vi "Reports.vi"() -> ()   [LabVIEW 2017]
uses:
  Globle/Breakdown Rep.vi
  Globle/Trigger Home Screen.vi
panel:
  out "appended array":refnum<vi>[](array[refnum])
  in  "Cancel Button\n- Archive":bool
  in  "Rej Cnt":bool
  in  "OEE":bool
  in  "PC Hr":bool
  in  "PC Day":bool
  in  "Para Report":bool
  in  "PC Month":bool
  in  "BD Day":bool
  in  "BD Yr":bool
  in  "BD Month":bool
  in  "BD MAnage":bool
  in  "BD Action Taken":bool
  in  "BD Analysis":bool
  # "Reports"
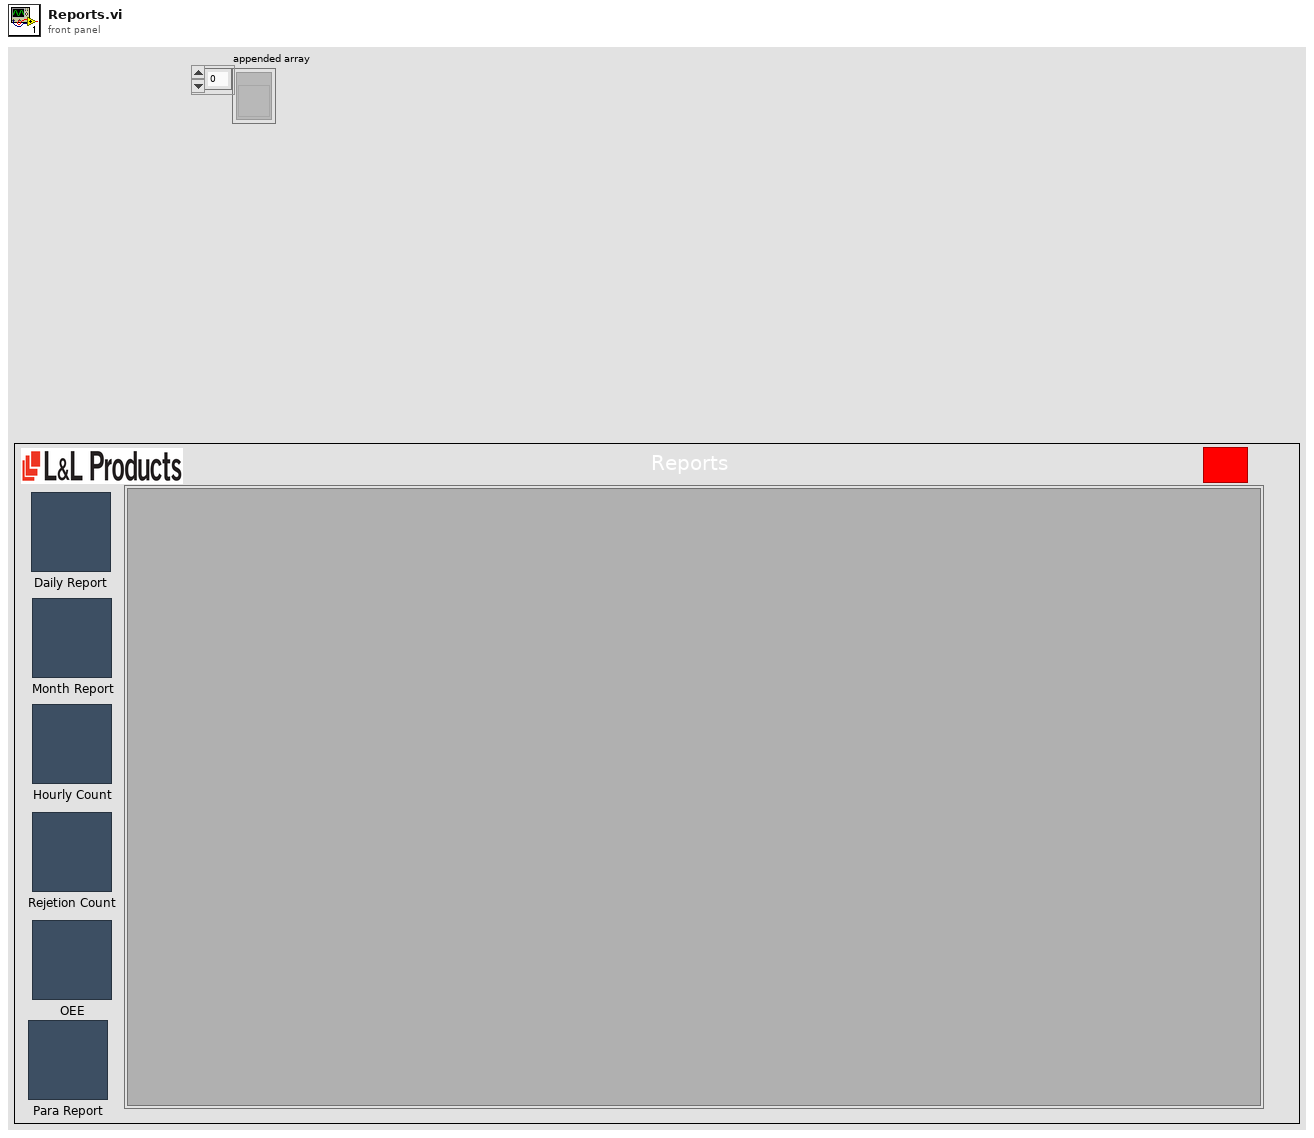
[diagram p1: front panel]
types:
  T1 = enum32{"invalid app kind", "Development System", "Run Time System", "Student Edition", "Embedded LabVIEW", "Evaluation", "Custom"}
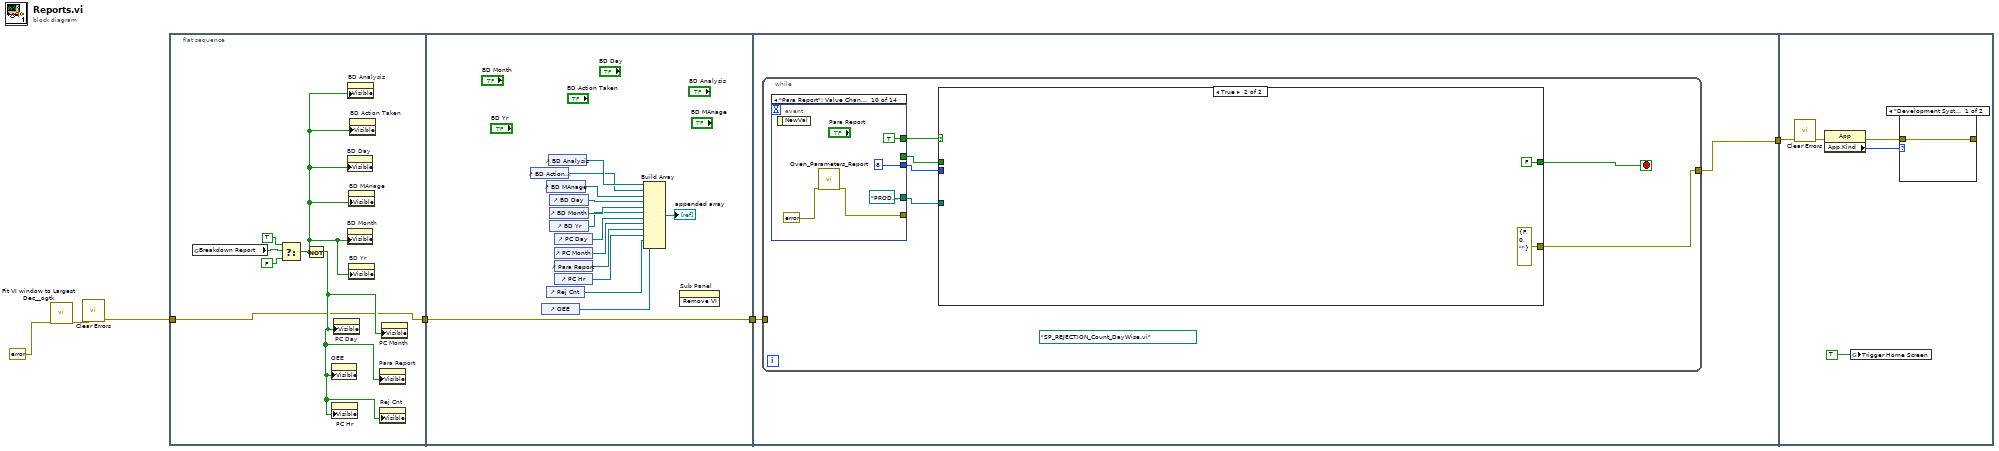
[diagram p0: block diagram]
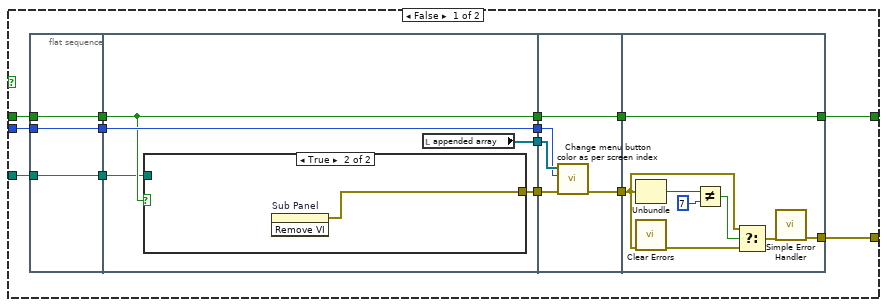
[diagram p2: hidden frame]
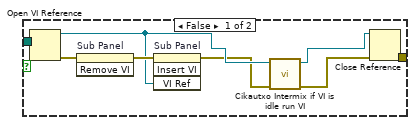
[diagram p3: hidden frame]
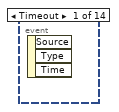
[diagram p4: hidden frame]
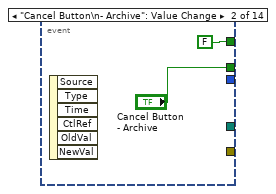
[diagram p5: hidden frame]
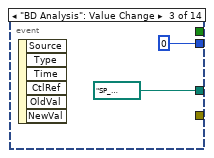
[diagram p6: hidden frame]
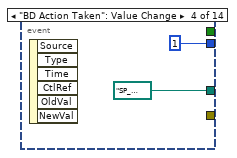
[diagram p7: hidden frame]
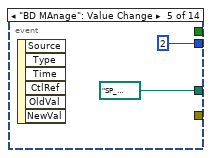
[diagram p8: hidden frame]
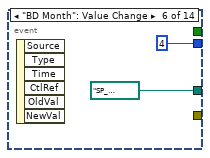
[diagram p9: hidden frame]
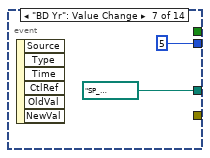
[diagram p10: hidden frame]
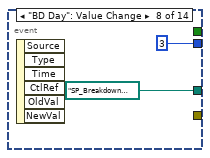
[diagram p11: hidden frame]
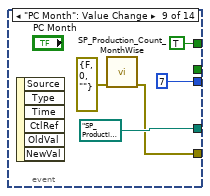
[diagram p12: hidden frame]
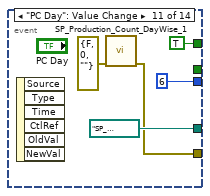
[diagram p13: hidden frame]
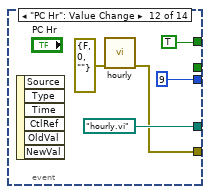
[diagram p14: hidden frame]
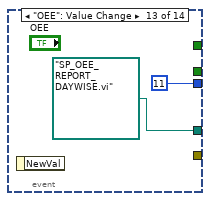
[diagram p15: hidden frame]
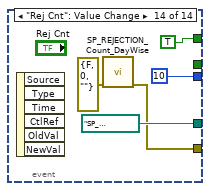
[diagram p16: hidden frame]
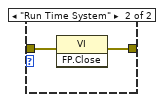
[diagram p17: hidden frame]
diagram:
  n1 = call <userlib>:"Fit VI window to Largest Dec__ogtk.vi"("error in (no error)"=errorcluster {"status"=FALSE, "code"=0, "source"=""}) -> ("error out"=w4:errorcluster)  [unwired: 5 in, 1 out]
  n2 = call <vilib>:"Clear Errors.vi"("error in (no error)"=w4) -> ("error out"=w3:errorcluster)  [unwired: 5 in, 1 out]
  n3 = flat-sequence {
    tunnel: w3 -> [w7]
    tunnel: [w7] -> w1
    tunnel: [w13] -> w2
    tunnel: w1 -> [w13]
    tunnel: [w28] -> w6
    tunnel: w2 -> [w27]
    tunnel: w6 -> [w123]
    frame #0 {
      n4 = global read "Breakdown Rep.vi" "Breakdown Report"() -> (w8:bool)
      n5 = Select(t=TRUE ("Visible"), s=w8, f=FALSE) -> (s? t:f=w10:bool)
      n6 = Not(x=w10) -> (.not. x?=w9:bool)
      n7 = property on="OEE" class="Bool"("Visible"=w9) -> ()  [unwired: 2 in, 2 out]
      n8 = property on="PC Hr" class="Bool"("Visible"=w9) -> ()  [unwired: 2 in, 2 out]
      n9 = property on="PC Day" class="Bool"("Visible"=w9) -> ()  [unwired: 2 in, 2 out]
      n10 = property on="BD Day" class="Bool"("Visible"=w10) -> ()  [unwired: 2 in, 2 out]
      n11 = property on="BD Month" class="Bool"("Visible"=w10) -> ()  [unwired: 2 in, 2 out]
      n12 = property on="BD Analysis" class="Bool"("Visible"=w10) -> ()  [unwired: 2 in, 2 out]
      n13 = property on="BD MAnage" class="Bool"("Visible"=w10) -> ()  [unwired: 2 in, 2 out]
      n14 = property on="BD Yr" class="Bool"("Visible"=w10) -> ()  [unwired: 2 in, 2 out]
      n15 = property on="BD Action Taken" class="Bool"("Visible"=w10) -> ()  [unwired: 2 in, 2 out]
      n16 = property on="Para Report" class="Bool"("Visible"=w9) -> ()  [unwired: 2 in, 2 out]
      n17 = property on="Rej Cnt" class="Bool"("Visible"=w9) -> ()  [unwired: 2 in, 2 out]
      n18 = property on="PC Month" class="Bool"("Visible"=w9) -> ()  [unwired: 2 in, 2 out]
    }
    frame #1 {
      n19 = control-ref of="BD Action Taken"() -> (w25:refnum<vi>)
      n20 = control-ref of="OEE"() -> (w15:refnum<vi>)
      n21 = control-ref of="Rej Cnt"() -> (w16:refnum<vi>)
      n22 = control-ref of="BD MAnage"() -> (w24:refnum<vi>)
      n23 = control-ref of="BD Analysis"() -> (w26:refnum<vi>)
      n24 = control-ref of="BD Day"() -> (w23:refnum<vi>)
      n25 = control-ref of="BD Month"() -> (w22:refnum<vi>)
      n26 = control-ref of="BD Yr"() -> (w21:refnum<vi>)
      n27 = control-ref of="PC Day"() -> (w20:refnum<vi>)
      n28 = control-ref of="PC Month"() -> (w19:refnum<vi>)
      n29 = control-ref of="Para Report"() -> (w18:refnum<vi>)
      n30 = control-ref of="PC Hr"() -> (w17:refnum<vi>)
      n31 = Build Array(w26, w25, w24, w23, w22, w21, w20, w19, w18, w17, w16, w15) -> (→"appended array":refnum<vi>[])
      n32 = invoke on="Sub Panel" class="SubPnl" method="Remove VI"() -> ()  [unwired: 3 in, 3 out]
    }
    frame #2 {
      n33 = while {
        tunnel: [w33] -> w28
        tunnel: w27 -> [_]
        stop <- w34 stop-if-true
        (unwired) path "SP_REJECTION_Count_DayWise.vi" ("vi path")
        n34 = event shown="[9] \"Para Report\": Value Change" {
          selector: _ -> [_ _ _ _ _ _ _ _ _ _ _ _ _ _]
          dyn-events: _ -> [_ _ _ _ _ _ _ _ _ _ _ _ _ _]
          timeout: _ -> [_ _ _ _ _ _ _ _ _ _ _ _ _ _]
          tunnel: [_ "Cancel Button\n- Archive" _ _ _ _ _ _ _ _ _ _ _ _] -> w31
          tunnel: [_ _ path "SP_Breakdown_Analysis.vi" ("vi path") path "SP_Action_Taken_Report.vi" ("vi path") path "SP_BreakDown_Manage.vi" ("vi path") path "SP_Breakdown Summery Monthwise_.vi" ("vi path") path "SP_Breakdown Summery Yearwise_.vi" ("vi path") path "SP_Breakdown Summery DayWisewise.vi" ("vi path") path "SP_Production_Count_MonthWise.vi" ("vi path") path "PRODUCTION_YEAR_main.vi" ("vi path") path "SP_Production_Count_DayWise_1.vi" ("vi path") path "hourly.vi" ("vi path") path "SP_OEE_REPORT_DAYWISE.vi" ("vi path") path "SP_REJECTION_Count_DayWise.vi" ("vi path")] -> w32
          tunnel: [_ _ 0 1 2 4 5 3 7 8 6 9 11 10] -> w30
          tunnel: [_ FALSE _ _ _ _ _ _ TRUE TRUE TRUE TRUE _ TRUE] -> w29
          tunnel: [_ _ _ _ _ _ _ _ w96 w100 w105 w111 _ w117] -> _
          event Timeout {
            n35 = event-data() -> ()  [unwired: 1 in, 3 out]
          }
          event "Cancel Button\n- Archive": Value Change {
            n36 = event-data() -> ()  [unwired: 1 in, 6 out]
          }
          event "BD Analysis": Value Change {
            n37 = event-data() -> ()  [unwired: 1 in, 6 out]
          }
          event "BD Action Taken": Value Change {
            n38 = event-data() -> ()  [unwired: 1 in, 6 out]
          }
          event "BD MAnage": Value Change {
            n39 = event-data() -> ()  [unwired: 1 in, 6 out]
          }
          event "BD Month": Value Change {
            n40 = event-data() -> ()  [unwired: 1 in, 6 out]
          }
          event "BD Yr": Value Change {
            n41 = event-data() -> ()  [unwired: 1 in, 6 out]
          }
          event "BD Day": Value Change {
            n42 = event-data() -> ()  [unwired: 1 in, 6 out]
          }
          event "PC Month": Value Change {
            n43 = event-data() -> ()  [unwired: 1 in, 6 out]
            n44 = call "SP_Production_Count_MonthWise.vi"("error in (no error)"=errorcluster {"status"=FALSE, "code"=0, "source"=""}) -> ("error out"=w96:errorcluster)  [unwired: 10 in]
          }
          event "Para Report": Value Change {
            n45 = event-data() -> ()  [unwired: 1 in, 1 out]
            n46 = call "Oven_Parameters_Report.vi"("error in (no error)"=errorcluster {"status"=FALSE, "code"=0, "source"=""}) -> ("error out"=w100:errorcluster)  [unwired: 10 in]
          }
          event "PC Day": Value Change {
            n47 = event-data() -> ()  [unwired: 1 in, 6 out]
            n48 = call "SP_Production_Count_DayWise_1.vi"("error in (no error)"=errorcluster {"status"=FALSE, "code"=0, "source"=""}) -> ("error out"=w105:errorcluster)  [unwired: 10 in]
          }
          event "PC Hr": Value Change {
            n49 = event-data() -> ()  [unwired: 1 in, 6 out]
            n50 = call "hourly.vi"("error in (no error)"=errorcluster {"status"=FALSE, "code"=0, "source"=""}) -> ("error out"=w111:errorcluster)  [unwired: 10 in]
          }
          event "OEE": Value Change {
            n51 = event-data() -> ()  [unwired: 1 in, 1 out]
          }
          event "Rej Cnt": Value Change {
            n52 = event-data() -> ()  [unwired: 1 in, 6 out]
            n53 = call "SP_REJECTION_Count_DayWise.vi"("error in (no error)"=errorcluster {"status"=FALSE, "code"=0, "source"=""}) -> ("error out"=w117:errorcluster)  [unwired: 10 in]
          }
        }
        n54 = case shown="True" w29 {
          tunnel: [w39 FALSE ("Cancel Button\n- Archive")] -> w34
          tunnel: [w38 errorcluster {"status"=FALSE, "code"=0, "source"=""} ("error out")] -> w33
          tunnel: w32 -> [w37 _]
          tunnel: w31 -> [w36 _]
          tunnel: w30 -> [w35 _]
          frame False {
            n55 = flat-sequence {
              tunnel: [w50] -> w48
              tunnel: [w51] -> w47
              tunnel: [w49] -> w46
              tunnel: w37 -> [w51]
              tunnel: w36 -> [w50]
              tunnel: w35 -> [w49]
              tunnel: w48 -> [w53]
              tunnel: w47 -> [w52]
              tunnel: [w53] -> w45
              tunnel: [w56] -> w44
              tunnel: [w55] -> w43
              tunnel: [w54] -> w42
              tunnel: w46 -> [w54]
              tunnel: w45 -> [w70]
              tunnel: [w70] -> w41
              tunnel: w44 -> [w69]
              tunnel: [w68] -> w40
              tunnel: w43 -> [w67]
              tunnel: w42 -> [w66]
              tunnel: [w78] -> w39
              tunnel: w41 -> [w78]
              tunnel: w40 -> [w71]
              tunnel: [w72] -> w38
              frame #0 {
              }
              frame #1 {
                n56 = case shown="True" w53 {
                  tunnel: w52 -> [w64 _]
                  tunnel: [w63 w65] -> w56
                  frame False {
                    n57 = Open VI Reference(vi path=w64) -> (vi reference=w60:refnum<vi>, error out=w62:errorcluster)  [unwired: 5 in]
                    n58 = invoke on="Sub Panel" class="SubPnl" method="Remove VI"(error in=w62) -> (error out=w61:errorcluster)  [unwired: 2 in, 2 out]
                    n59 = invoke on="Sub Panel" class="SubPnl" method="Insert VI"(error in=w61, "VI Ref"=w60) -> (error out=w58:errorcluster)  [unwired: 2 in, 3 out]
                    n60 = call "Cikautxo Intermix if VI is idle run VI.vi"("error in (no error)"=w58, "VI in"=w60) -> ("error out"=w57:errorcluster, "VI out"=w59:refnum<vi>)  [unwired: 8 in]
                    n61 = Close Reference(reference=w59, error in (no error)=w57) -> (error out=w63:errorcluster)
                  }
                  frame True {
                    n62 = invoke on="Sub Panel" class="SubPnl" method="Remove VI"() -> (error out=w65:errorcluster)  [unwired: 3 in, 2 out]
                  }
                }
                n63 = local read "appended array"() -> (w55:refnum<vi>[])
              }
              frame #2 {
                n64 = call "Change menu button color as per screen index.vi"("error in (no error)"=w69, "Screen Index"=w66, "Array"=w67) -> ("error out"=w68:errorcluster)  [unwired: 8 in]
              }
              frame #3 {
                n65 = Unbundle(w71) -> ("code"=w77:i32)  [unwired: 2 out]
                n66 = call <vilib>:"Clear Errors.vi"("error in (no error)"=w71) -> ("error out"=w74:errorcluster)  [unwired: 5 in, 1 out]
                n67 = Not Equal?(x=w77, y=7) -> (x != y?=w75:bool)
                n68 = Select(t=w71, s=w75, f=w74) -> (s? t:f=w73:errorcluster)
                n69 = call <vilib>:"Simple Error Handler.vi"("error in (no error)"=w73) -> ("error out"=w72:errorcluster)  [unwired: 4 in, 4 out]
              }
            }
          }
          frame True {
          }
        }
      }
    }
    frame #3 {
      n70 = call <vilib>:"Clear Errors.vi"("error in (no error)"=w123) -> ("error out"=w126:errorcluster)  [unwired: 5 in, 1 out]
      n71 = property class="App"(error in=w126) -> (error out=w125:errorcluster, "App.Kind"=w124:T1)  [unwired: 1 in, 1 out]
      n72 = global write "Trigger Home Screen.vi" "Trigger Home Screen"(TRUE ("Trigger Home Screen")) -> ()
      n73 = case shown="\"Development System\", Default" w124 {
        tunnel: w125 -> [w127 w129]
        tunnel: [w127 w128] -> _
        frame "Development System", Default {
        }
        frame "Run Time System" {
          n74 = invoke class="VI" method="FP.Close"(error in=w129) -> (error out=w128:errorcluster)  [unwired: 2 in, 2 out]
        }
      }
    }
  }
